vi "Vertical Mirror.vi"(7 "N":i32, 10 "Mirror Position":i32, 11 "Rocks":cluster{i32, i32}[](array[cluster])) -> (2 "Mirror?":bool, 3 "Mirrored Columns":u64)   [LabVIEW 2023, in "d13.lvlib"]
uses:
  d13.lvlib
  b04d7152-596d-4885-9dda-5841b427e0d8.vi
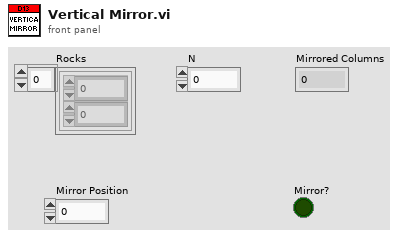
[diagram p1: front panel]
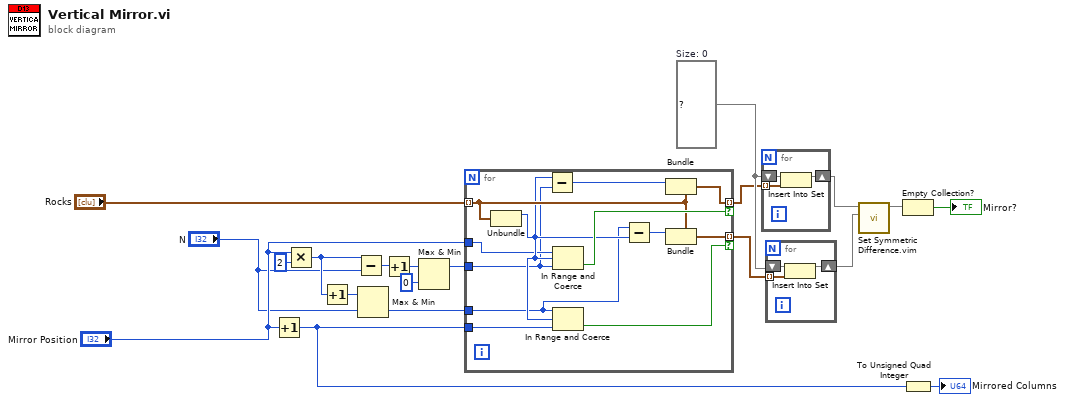
[diagram p0: block diagram]
diagram:
  w18 = set{cluster{"offset of match":i32, i32}} {}  # Size: 0
  n1 = Increment(x="Mirror Position") -> (x+1=w6:i32)
  n2 = Multiply(x="Mirror Position", y=2) -> (x*y=w10:i32)
  n3 = Increment(x=w10) -> (x+1=w7:i32)
  n4 = Subtract(x=w10, y="N") -> (x-y=w13:i32)
  n5 = Max & Min(x=w7, y="N") -> (min(x,y)=w9:i32)  [unwired: 1 out]
  n6 = Increment(x=w13) -> (x+1=w12:i32)
  n7 = Max & Min(x=w12, y=0) -> (max(x,y)=w11:i32)  [unwired: 1 out]
  n8 = for {
    tunnel: "Rocks" -> [w28] mode=indexing
    tunnel: [w27] -> w16 mode=indexing if=w30
    tunnel: [w32] -> w8 mode=indexing if=w31
    tunnel: w11 -> [w23]
    tunnel: "Mirror Position" -> [w24]
    tunnel: w6 -> [w22]
    tunnel: w9 -> [w21]
    n9 = Unbundle(w28) -> (w26:i32)  [unwired: 1 out]
    n10 = Subtract(x=w26, y=w23) -> (x-y=w25:i32)
    n11 = In Range and Coerce(upper limit=w24, x=w26, lower limit=w23) -> (In Range?=w30:bool)  [unwired: 1 out]
    n12 = In Range and Coerce(upper limit=w21, x=w26, lower limit=w22) -> (In Range?=w31:bool)  [unwired: 1 out]
    n13 = Subtract(x=w21, y=w26) -> (x-y=w29:i32)
    n14 = Bundle(cluster=w28, w25) -> (w27:cluster{i32, i32})  [unwired: 1 in]
    n15 = Bundle(cluster=w28, w29) -> (w32:cluster{i32, i32})  [unwired: 1 in]
  }
  n16 = for {
    tunnel: w16 -> [w35] mode=indexing
    shift-right: [w33] -> w5
    shift-left: w18 -> [w34]
    n17 = Insert Into Set(10:w35, 11:w34) -> (3:w33:set{cluster{"offset of match":i32, i32}})  [unwired: 1 out]
  }
  n18 = for {
    tunnel: w8 -> [w38] mode=indexing
    shift-right: [w36] -> w4
    shift-left: w18 -> [w37]
    n19 = Insert Into Set(10:w38, 11:w37) -> (3:w36:set{cluster{"offset of match":i32, i32}})  [unwired: 1 out]
  }
  n20 = call "Set Symmetric Difference.vim"("set 2"=w4, "set 1"=w5) -> ("symmetric difference"=w3:set{cluster{"offset of match":i32, i32}})  [unwired: 9 in]
  n21 = Empty Collection?(1:w3) -> (0:→"Mirror?":bool)
  n22 = To Unsigned Quad Integer(1:w6) -> (0:→"Mirrored Columns":u64)
